vi "Sandbox.vi"() -> ()   [LabVIEW 2017]
uses:
  <vilib>/NI/NonreentrantSinglePoint/Multiplier/Multiplier.lvclass
  <vilib>/NI/NonreentrantSinglePoint/Divider/Divider.lvclass
  <vilib>/NI/NonreentrantSinglePoint/Adder/Adder.lvclass
  <vilib>/NI/PowerElectronicsControl/Transforms/_IPBuilder/AlphaBetaAndDQ_variants/ABCtoAlphaBeta_3PhaseUnitaryMagnitude_src.vi
  SVPWM/SVPWM.lvlib
panel:
  in  "manual":bool
  in  "ref_beta":sgl
  in  "ref_alpha":sgl=0.1
  in  "ref_max":sgl=0.9999695 caption="max voltage"
  out "Waveform Chart":dbl[][](graph)
  in  "speed":u32=10
  out "Sector 6":bool
  out "Sector 5":bool
  out "Sector 4":bool
  out "Sector 3":bool
  out "Sector 2":bool
  out "Sector 1":bool
  out "Alpha-Beta":cluster{"X":dbl, "Y":dbl}[](graph)
  in  "modulation":dbl=1.0 format="%#_13g"
  in  "stop":bool
  # "[0, Vdc, 0]"
  # "[Vdc, Vdc, 0]"
  # "[0%, Vdc, Vdc]"
  # "[100%, 0%, 0%]"
  # "[0, 0, Vdc]"
  # "[Vdc, 0, Vdc]"
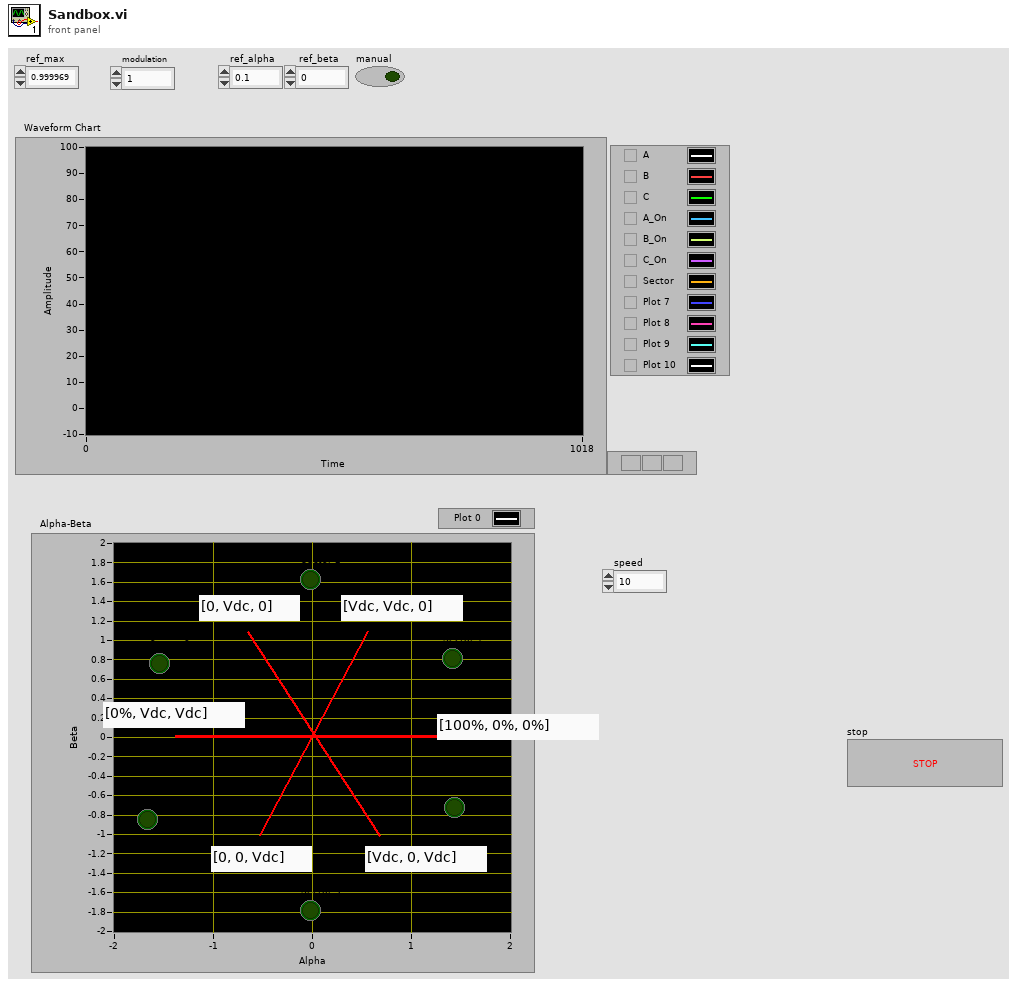
[diagram p1: front panel]
types:
  T1 = cluster{"Multiplier":refnum<class "Multiplier.lvclass">, "Divider":refnum<class "Divider.lvclass">, "Adder":refnum<class "Adder.lvclass">}
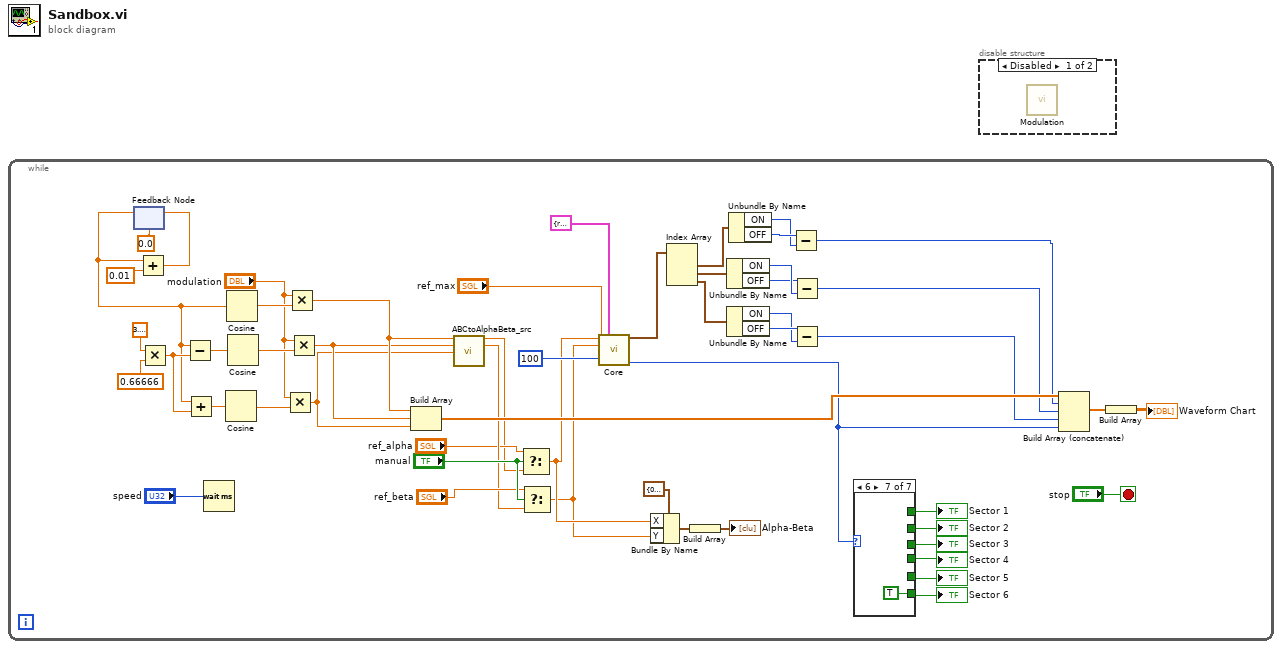
[diagram p0: block diagram]
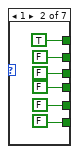
[diagram p4: hidden frame]
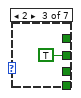
[diagram p5: hidden frame]
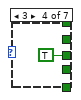
[diagram p6: hidden frame]
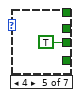
[diagram p7: hidden frame]
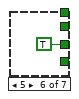
[diagram p8: hidden frame]
diagram:
  n1 = while {
    stop <- "stop" stop-if-true
    n2 = feedback #1(0.0) -> (w40:dbl)
    n3 = Add(x=w40, y=0.01) -> (x+y=w42:dbl)
    n4 = feedback-in #1(w42) -> ()
    n5 = Multiply(x=3.141592653589793, y=0.66666) -> (x*y=w51:dbl)
    n6 = Subtract(x=w40, y=w51) -> (x-y=w50:dbl)
    n7 = Add(x=w40, y=w51) -> (x+y=w49:dbl)
    n8 = Wait (ms)(milliseconds to wait="speed") -> ()  [unwired: 1 out]
    n9 = Cosine(x=w49) -> (cos(x)=w44:dbl)
    n10 = Cosine(x=w40) -> (cos(x)=w46:dbl)
    n11 = Cosine(x=w50) -> (cos(x)=w45:dbl)
    n12 = Multiply(x="modulation", y=w44) -> (x*y=w28:dbl)
    n13 = Multiply(x="modulation", y=w46) -> (x*y=w30:dbl)
    n14 = Multiply(x="modulation", y=w45) -> (x*y=w29:dbl)
    n15 = Build Array(w30, w29, w28) -> (w27:dbl[])
    n16 = call-poly <vilib>:"ABCtoAlphaBeta_src.vi"("A"=w30, "B"=w29, "C"=w28) -> ("alpha"=w16:sgl, "beta"=w18:sgl)  [unwired: 11 in]
    n17 = Select(t="ref_alpha", s="manual", f=w16) -> (s? t:f=w21:sgl)
    n18 = Select(t="ref_beta", s="manual", f=w18) -> (s? t:f=w15:sgl)
    n19 = call "Core.vi"("ref_alpha"=w21, "Resource"=T1 {"Multiplier"=refnum, "Divider"=refnum, "Adder"=refnum}, "ref_beta"=w15, "ref_max"="ref_max", "Period"=u32 100) -> ("SVPWM_Timing"=w5:cluster{"ON":u32, "OFF":u32}[], "SVPWM_Sector"=w26:u8)  [unwired: 9 in]
    n20 = Bundle By Name(cluster=cluster{"X":dbl, "Y":dbl} {"X"=0.0, "Y"=0.0}, "X"=w21, "Y"=w15) -> (w38:cluster{"X":dbl, "Y":dbl})
    n21 = Index Array(array=w5) -> (element #1=w4:cluster{"ON":u32, "OFF":u32}, element #2=w3:cluster{"ON":u32, "OFF":u32}, element #3=w2:cluster{"ON":u32, "OFF":u32})  [unwired: 3 in]
    n22 = Build Array(w38) -> (→"Alpha-Beta":cluster{"X":dbl, "Y":dbl}[])
    n23 = Unbundle By Name(w3) -> ("ON"=w14:u32, "OFF"=w13:u32)
    n24 = Unbundle By Name(w2) -> ("ON"=w11:u32, "OFF"=w12:u32)
    n25 = Unbundle By Name(w4) -> ("ON"=w7:u32, "OFF"=w8:u32)
    n26 = Subtract(x=w8, y=w7) -> (x-y=w6:u32)
    n27 = Subtract(x=w13, y=w14) -> (x-y=w10:u32)
    n28 = Subtract(x=w12, y=w11) -> (x-y=w9:u32)
    n29 = case shown="6" w26 {
      tunnel: [_ TRUE ("Sector 1") _ _ _ _ _] -> w36
      tunnel: [_ FALSE ("Sector 2") TRUE ("Sector 2") _ _ _ _] -> w35
      tunnel: [_ FALSE ("Sector 3") _ TRUE ("Sector 3") _ _ _] -> w34
      tunnel: [_ FALSE ("Sector 4") _ _ TRUE ("Sector 4") _ _] -> w33
      tunnel: [_ FALSE ("Sector 5") _ _ _ TRUE ("Sector 5") _] -> w32
      tunnel: [_ FALSE ("Sector 6") _ _ _ _ TRUE ("Sector 6")] -> w31
      frame Default {
      }
      frame 1 {
      }
      frame 2 {
      }
      frame 3 {
      }
      frame 4 {
      }
      frame 5 {
      }
      frame 6 {
      }
    }
    "Sector 1" <- w36
    "Sector 2" <- w35
    "Sector 3" <- w34
    "Sector 4" <- w33
    "Sector 5" <- w32
    "Sector 6" <- w31
    n30 = Build Array (concatenate)(w27, w6, w10, w9, w26) -> (w25:dbl[])
    n31 = Build Array(w25) -> (→"Waveform Chart":dbl[][])
  }
  n32 = disable-structure shown="Disabled" {
    frame Disabled {
      n33 = call "Modulation.vi"() -> ()  [unwired: 15 in, 1 out]
    }
    frame Enabled {
    }
  }
